vi "Shilong_Smoothing.vi"(6 "GetPoint":dbl=1.0, 8 "1-D Array of Real  Source":dbl[](array[numeric])=[10.0, 10.0, 10.0, 20.0, 20.0, 20.0, 20.0, 20.0, 30.0, 12.36, 54.21, 12.56, 148.21, 65.21, 1.2, 35.14, 47.02, 20.0, 32.21, 21.36, 21.32, 21.36, 21.21, 41.32, 24.12]) -> (3 "子数组":dbl[](array[numeric]))   [LabVIEW 2011]
panel:
  out "波形图":dbl[](graph)
  out "Source 波形图":dbl[](graph)
  out "2-D Array of Real  After Smooth":dbl[][](array[numeric])
  # "Smoothing Functon  VI"
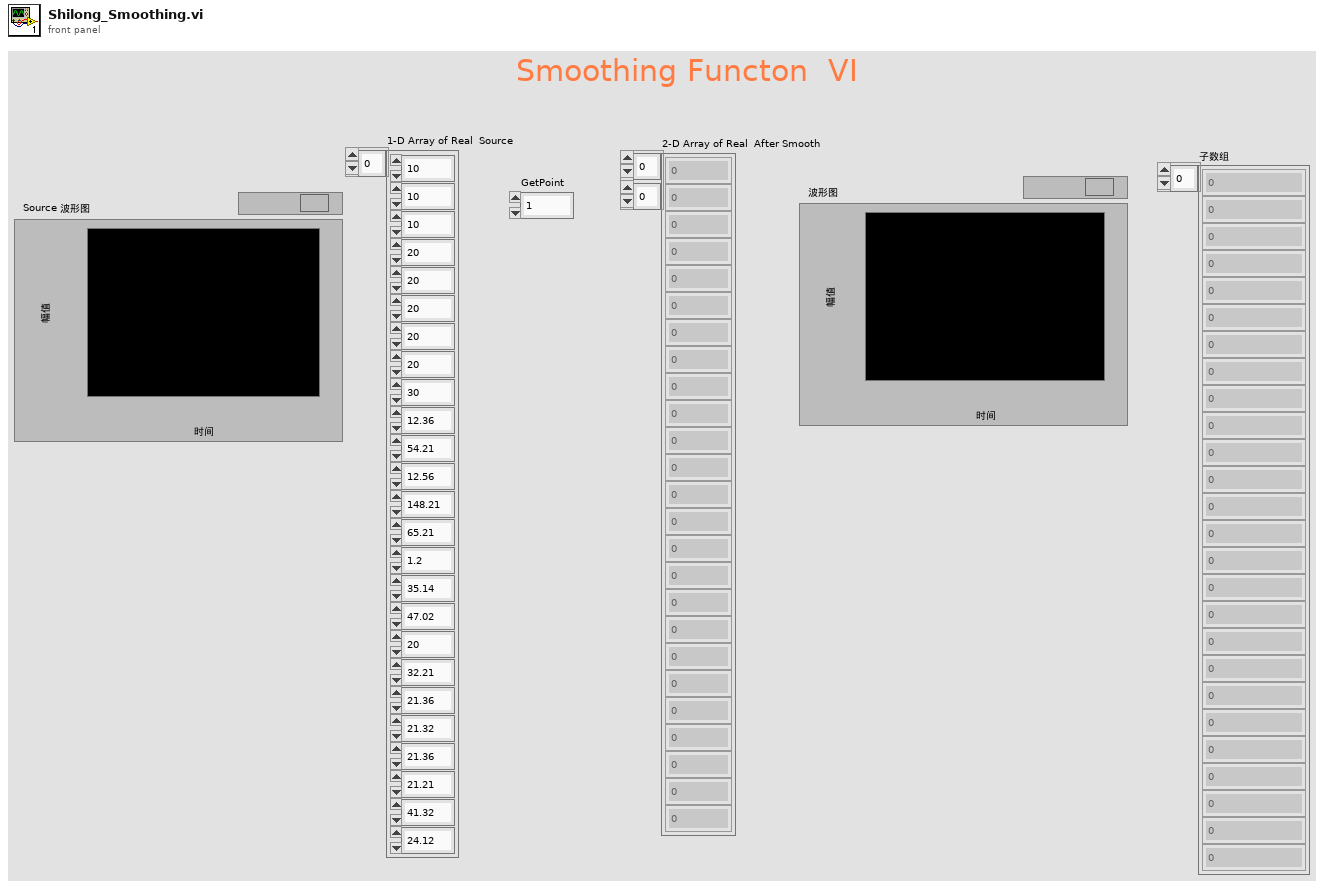
[diagram p1: front panel]
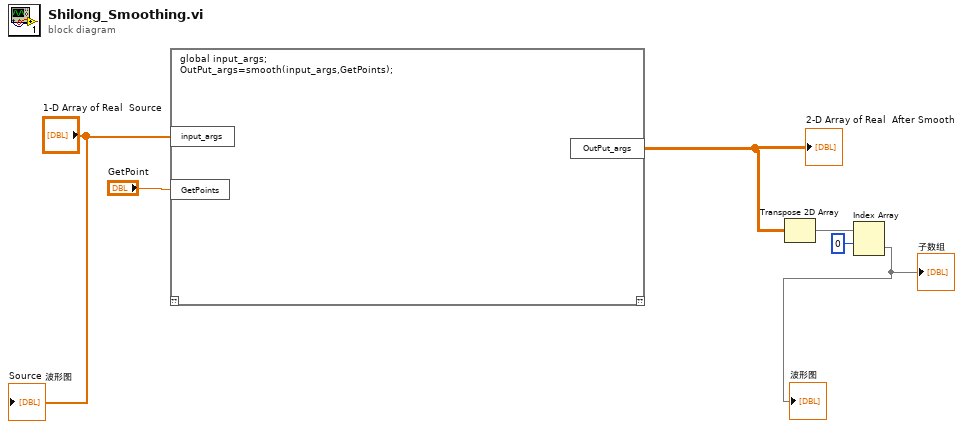
[diagram p0: block diagram]
diagram:
  n1 = script code="global input_args;\nOutPut_args=smooth(input_args,GetPoints);"("input_args"="1-D Array of Real  Source", "GetPoints"="GetPoint") -> ("OutPut_args"=w4:dbl[][])  [unwired: 1 in, 1 out]
  "2-D Array of Real  After Smooth" <- w4
  n2 = Transpose 2D Array(2D array=w4) -> (transposed array=w3:dbl[][])
  n3 = Index Array(array=w3, index (row)=0 ("索引 (行)")) -> (element=→"波形图" →"子数组":dbl[])  [unwired: 1 in]
  "Source 波形图" <- "1-D Array of Real  Source"
